vi "Extractvalue.vi"(1 "Chaîne":string) -> (0 "Numeric":dbl)   [LabVIEW 2018]
panel:
  in  "Chaîne 2":string
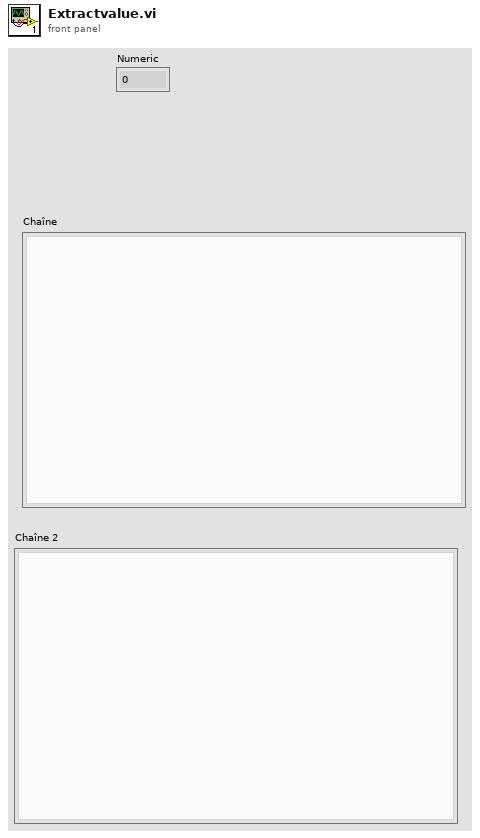
[diagram p1: front panel]
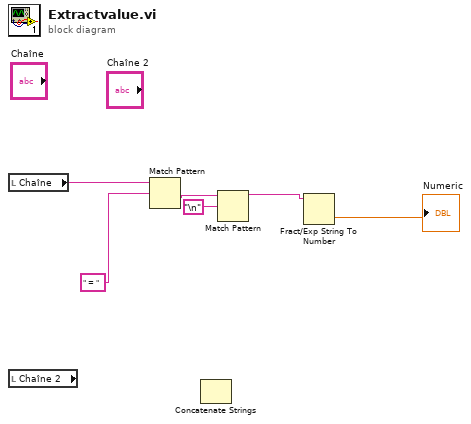
[diagram p0: block diagram]
diagram:
  n1 = local read "Chaîne"() -> (w6:string)
  n2 = local read "Chaîne 2"() -> ()  [unwired: 1 out]
  n3 = Match Pattern(string=w6, regular expression=" = ") -> (after substring=w4:string)  [unwired: 1 in, 3 out]
  n4 = Concatenate Strings() -> ()  [unwired: 3 in, 1 out]
  n5 = Match Pattern(string=w4, regular expression="\n") -> (before substring=w2:string)  [unwired: 1 in, 3 out]
  n6 = Fract/Exp String To Number(string=w2) -> (number=→"Numeric":dbl)  [unwired: 3 in, 1 out]
